vi "Match Number.vi"() -> ()   [LabVIEW 2014]
panel:
  out "# itterations":dbl
  out "Current number":dbl
  in  "number to match":dbl min=0.0 max=10000.0 step=1.0
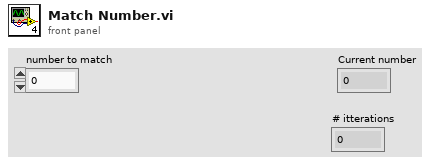
[diagram p1: front panel]
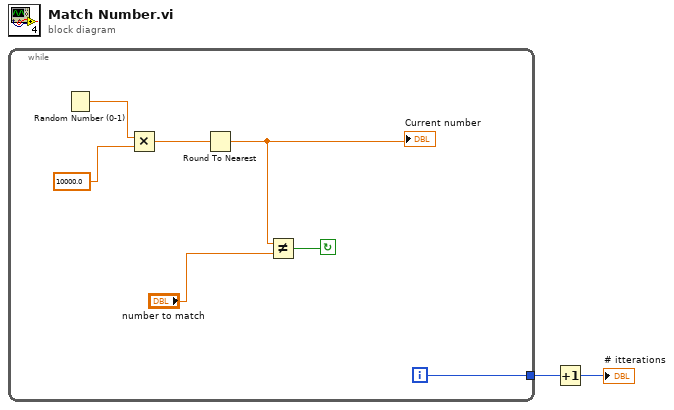
[diagram p0: block diagram]
diagram:
  n1 = while {
    tunnel: [w3] -> w1
    i -> [w3]
    stop <- w4 continue-if-true
    n2 = Random Number (0-1)() -> (number: 0 to 1=w9:dbl)
    n3 = Multiply(x=w9, y=10000.0) -> (x*y=w7:dbl)
    n4 = Round To Nearest(number=w7) -> (nearest integer value=w5:dbl)
    "Current number" <- w5
    n5 = Not Equal?(x=w5, y="number to match") -> (x != y?=w4:bool)
  }
  n6 = Increment(x=w1) -> (x+1=→"# itterations":i32)
